vi "pzt test.vi"   [LabVIEW 2019]
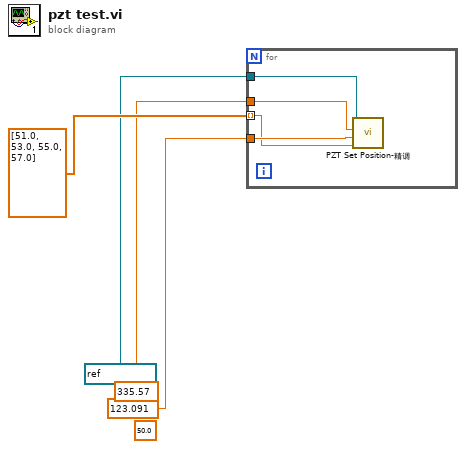
[diagram p0: block diagram]
diagram:
  (unwired) 50.0 ("Set Position （°/mm）")
  n1 = for {
    tunnel: dbl[] [51.0, 53.0, 55.0, 57.0] ("array") -> [w5] mode=indexing
    tunnel: 123.091 ("Origin") -> [w8]
    tunnel: 335.57 ("Range") -> [w7]
    tunnel: refnum<visa-resource-name> "COM12" ("VISA resource name") -> [w6]
    n2 = call "PZT Set Position-精调.vi"("Set Position （°/mm）"=w5, "Origin"=w8, "Range"=w7, "VISA resource name"=w6) -> ()  [unwired: 5 in, 3 out]
  }
